vi "Target Load Cell Read TB 4330 Two Load Cells.vi"(11 "task/channels in":refnum<k21>) -> (0 "Ankle Cable Force (N)":dbl, 3 "Knee Cable Force (N)":dbl)   [LabVIEW 2018, in "COBRA Measurement and Filtering Library.lvlib"]
uses:
  COBRA Measurement and Filtering Library.lvlib
  <vilib>/DAQmx/read.llb/DAQmx Read (Analog 1D DBL NChan 1Samp).vi
  <vilib>/DAQmx/configure/timing.llb/DAQmx Timing (Sample Clock).vi
  <vilib>/DAQmx/miscellaneous.llb/DAQmx Fill In Error Info.vi
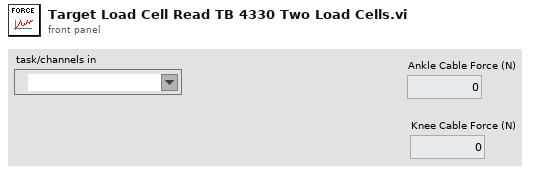
[diagram p1: front panel]
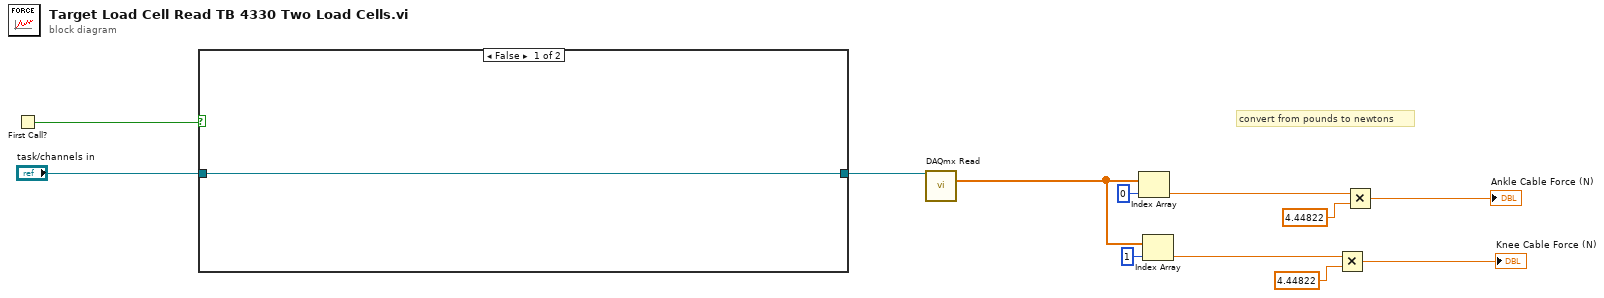
[diagram p0: block diagram]
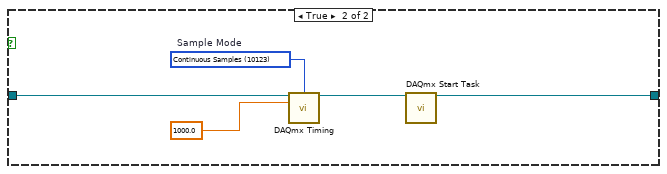
[diagram p2: hidden frame]
diagram:
  # "convert from pounds to newtons"
  n1 = First Call?() -> (First Call?: T/F=w8:bool)
  n2 = case shown="False" w8 {
    tunnel: "task/channels in" -> [w13 w16]
    tunnel: [w13 w18] -> w11
    frame False {
    }
    frame True {
      w17 = 10123 items=["Finite Samples"=10178, "Continuous Samples"=10123, "Hardware Timed Single Point"=12522]  # Sample Mode
      n3 = call-poly <vilib>:"DAQmx Timing.vi"("task/channels in"=w16, "sample mode"=w17, "rate"=1000.0) -> ("task out"=w15:refnum<k21>)  [unwired: 11 in, 1 out]
      n4 = call <vilib>:"DAQmx Start Task.vi"("task/channels in"=w15) -> ("task out"=w18:refnum<k21>)  [unwired: 13 in, 1 out]
    }
  }
  n5 = call-poly <vilib>:"DAQmx Read.vi"("task/channels in"=w11) -> ("data"=w5:dbl[])  [unwired: 12 in, 2 out]
  n6 = Index Array(array=w5, index=0) -> (element=w4:dbl)
  n7 = Index Array(array=w5, index=1) -> (element=w2:dbl)
  n8 = Multiply(x=w2, y=4.44822 ("Cable Force (N)")) -> (x*y=→"Knee Cable Force (N)":dbl)
  n9 = Multiply(x=w4, y=4.44822 ("Cable Force (N)")) -> (x*y=→"Ankle Cable Force (N)":dbl)
